vi "Parse Integer.vi"(8 "error in (no error)":errorcluster, 11 "Alpaca CLI Parser in":refnum<class "JSON Parser.lvclass">) -> (0 "error out":errorcluster, 2 "Value":variant, 3 "Alpaca CLI Parser out":refnum<class "JSON Parser.lvclass">)   [LabVIEW 2019, in "JKI JSON Serialization.lvlib" / "JSON Parser.lvclass"]
doc: "JKI JSON 1.1.10.37\nTomi Maila - JKI\nCopyright (c) 2017, JKI"
uses:
  JSON Parser.lvclass
  C:/Users/Patrick/Documents/GitHub/Instrument-Framework/lvsrc/SMOs/JSON-RPC-2019/lv-venv/lv.lib/vi.lib/addons/_JKI.lib/Serialization/JSON/Deserializer/Parser/Parser.lvclass
  Parser/Parser.lvclass/Parser.ctl
  Parser/Lookahead.vi
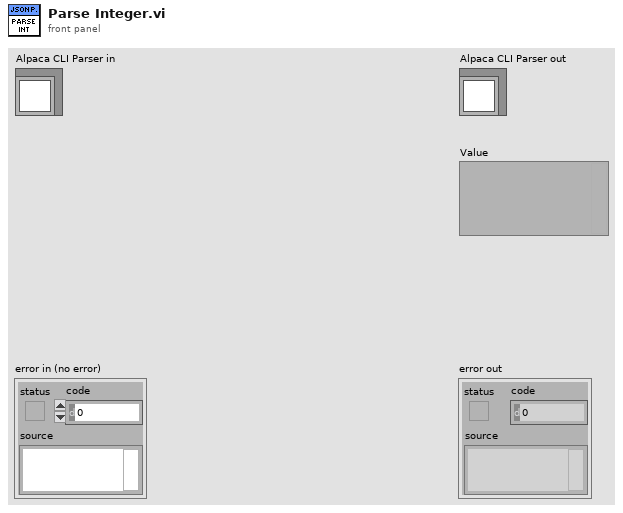
[diagram p1: front panel]
types:
  T1 = typedef "JKI JSON Serialization.lvlib/JSON Lexer.lvclass/JSON Token Type.ctl" = enum32{"unknown", "comma", "end-label", "begin-object", "end-object", "begin-array", "end-array", "quoted-string", "boolean", "exponential-number", "decimal-number", "integer-number", "special-number", "null", "symbol", "whitespace", "EOF"}
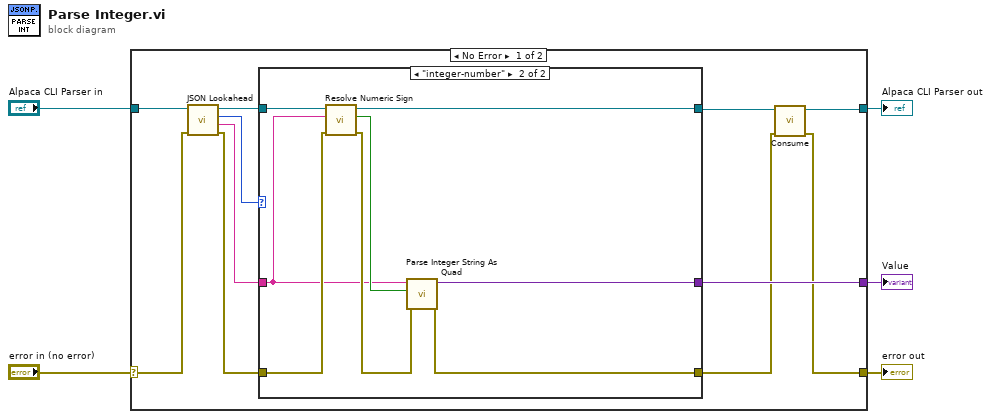
[diagram p0: block diagram]
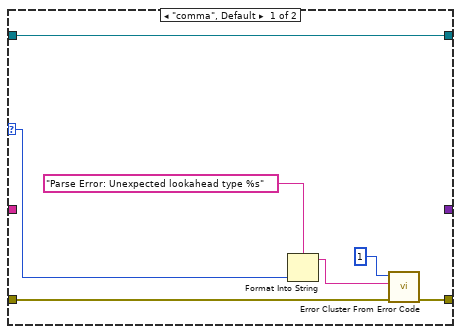
[diagram p2: hidden frame]
diagram:
  n1 = case shown="No Error" "error in (no error)" {
    selector: "error in (no error)" -> [w15 w33]
    tunnel: [w8 w33] -> w4
    tunnel: [w6 w32] -> w2
    tunnel: "Alpaca CLI Parser in" -> [w16 w32]
    tunnel: [w10 _] -> w1
    frame No Error {
      n2 = call "JSON Lookahead.vi"("error in (no error)"=w15, "Alpaca CLI Parser in"=w16) -> ("error out"=w12:errorcluster, "Lookahead Value"=w11:string, "Lookahead Type"=w13:T1, "Alpaca CLI Parser out"=w14:refnum<class "JSON Parser.lvclass">)  [unwired: 6 in]
      n3 = case shown="\"integer-number\"" w13 {
        selector: w13 -> [w19 _]
        tunnel: w14 -> [w17 w31]
        tunnel: [w17 w30] -> w9
        tunnel: [w23 w27] -> w7
        tunnel: w12 -> [w22 w29]
        tunnel: w11 -> [_ w24]
        tunnel: [_ w26] -> w10
        frame "comma", Default {
          n4 = Format Into String(format string="Parse Error: Unexpected lookahead type %s" ("error message (\"\")"), w19) -> (resulting string=w18:string)  [unwired: 2 in, 1 out]
          n5 = call <vilib>:"Error Cluster From Error Code.vi"("error in (no error)"=w22, "error message (\"\")"=w18, "error code (0)"=1) -> ("error out"=w23:errorcluster)  [unwired: 6 in]
        }
        frame "integer-number" {
          n6 = call-dynamic "Resolve Numeric Sign.vi"("error in (no error)"=w29, "Numeric String"=w24, "Alpaca CLI Parser in"=w31) -> ("error out"=w28:errorcluster, "Negative?"=w25:bool, "Alpaca CLI Parser out"=w30:refnum<class "JSON Parser.lvclass">)  [unwired: 6 in]
          n7 = call "Parse Integer String As Quad.vi"("error in (no error)"=w28, "Negative"=w25, "String"=w24) -> ("error out"=w27:errorcluster, "Value"=w26:variant)  [unwired: 7 in]
        }
      }
      n8 = call-dynamic "Consume.vi"("error in (no error)"=w7, "Alpaca Parser in"=w9) -> ("error out"=w8:errorcluster, "Alpaca Parser out"=w6:refnum<class "JSON Parser.lvclass">)  [unwired: 8 in]
    }
    frame Error {
    }
  }
  "error out" <- w4
  "Alpaca CLI Parser out" <- w2
  "Value" <- w1
